vi "Get Master Bounds Rect.vi"(8 "error in (no error)":errorcluster, 11 "Object Layout in":refnum<class "Object Layout.lvclass">) -> (0 "error out":errorcluster, 2 "Rect":T1, 3 "Object Layout out":refnum<class "Object Layout.lvclass">)   [LabVIEW 2012, in "NI_SE_Front Panel Layout.lvlib" / "Object Layout.lvclass"]
uses:
  Object Layout.lvclass
  <vilib>/Utility/miscctls.llb/LVRectTypeDef.ctl
  Object Layout.lvclass/Object Layout.ctl
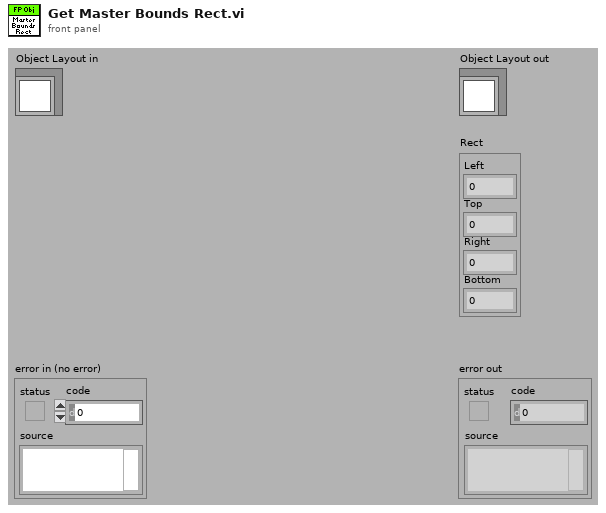
[diagram p1: front panel]
types:
  T1 = typedef "LVRectTypeDef.ctl" = cluster{"Left":i16, "Top":i16, "Right":i16, "Bottom":i16}
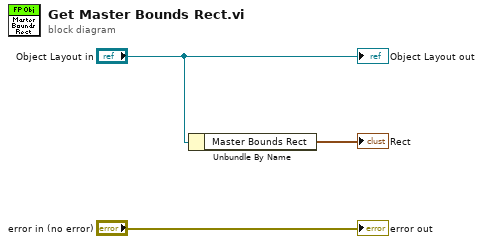
[diagram p0: block diagram]
diagram:
  n1 = Unbundle By Name("Object Layout in") -> ("Master Bounds Rect"=→"Rect":T1)
  "error out" <- "error in (no error)"
  "Object Layout out" <- "Object Layout in"
